vi "Do.vi"(8 "error in (no error)":errorcluster, 10 "Actor in":refnum<class "Actor.lvclass">, 11 "Set Ratios Msg":refnum<class "Set Ratios Msg.lvclass">) -> (0 "error out":errorcluster, 2 "Actor out":refnum<class "Actor.lvclass">)   [LabVIEW 2020, in "BNT_ULx.lvlib" / "Set Ratios Msg.lvclass"]
doc: "This VI delivers the message to the actor by calling the appropriate method(s) on the actor."
uses:
  Set Ratios Msg.lvclass
  <vilib>/ActorFramework/Actor/Actor.lvclass
  C:/User/Brand/LVP/CSPP/CSPP-Template/Packages/CSPP_Core/Messages/CSPP_PVUpdate Msg/CSPP_PVUpdate Msg.lvclass
  BNT_ULx-MCSV-DOPWM/BNT_ULx-MCSV-DOPWM.lvclass
  C:/Program Files (x86)/National Instruments/LabVIEW 2020/vi.lib/ActorFramework/Actor/Actor.lvclass
  CSPP_Core/Messages/CSPP_PVUpdate Msg/CSPP_PVUpdate Msg.lvclass/CSPP_PVUpdate Msg.ctl
  CSPP_Core/Classes/CSPP_ProcessVariables/ProcessVariable/PV.lvclass/PV.ctl
  Set Ratios Msg.lvclass/Set Ratios Msg.ctl
  CSPP_Core/Classes/CSPP_ProcessVariables/ProcessVariable/PV.lvclass
  CSPP_Core/Messages/CSPP_PVUpdate Msg/CSPP_PVUpdate Msg.lvclass
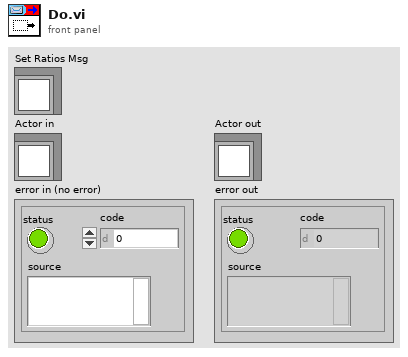
[diagram p1: front panel]
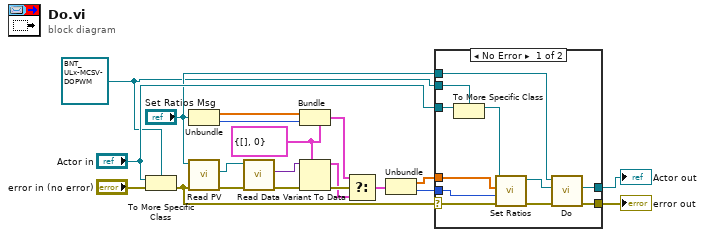
[diagram p0: block diagram]
diagram:
  w1 = refnum<class "BNT_ULx-MCSV-DOPWM.lvclass"> refnum ("BNT_ULx.lvlib:BNT_ULx-MCSV-DOPWM.lvclass")
  w14 = cluster{"PWM Ratios":dbl[], "Start Index":i32} {"PWM Ratios"=[], "Start Index"=0} ("Type")
  n1 = To More Specific Class(target class=w1, reference="Actor in", error in="error in (no error)") -> (error out=w11:errorcluster)  [unwired: 1 out]
  n2 = Unbundle ("Pre-Unbundler")("Set Ratios Msg") -> (w3:dbl[], w2:i32)
  n3 = call "Read PV.vi"("error in (no error)"=w11, "CS++PVUpdate Msg in"="Set Ratios Msg") -> ("error out"=w16:errorcluster, "PV"=w13:refnum<class "PV.lvclass">)  [unwired: 7 in, 1 out]
  n4 = call "Read Data.vi"("error in (no error)"=w16, "PV in"=w13) -> ("error out"=w7:errorcluster, "Data"=w6:variant)  [unwired: 7 in, 1 out]
  n5 = Bundle ("Pre-Bundler")(cluster=w14, "PWM Ratios"=w3, "Start Index"=w2) -> (w8:cluster{"PWM Ratios":dbl[], "Start Index":i32})
  n6 = Variant To Data(error in=w7, type=w14, Variant=w6) -> (data=w9:cluster{"PWM Ratios":dbl[], "Start Index":i32}, error out=w15:errorcluster)
  n7 = Select ("MainSelect")(t=w8, s=w15, f=w9) -> (s? t:f=w12:cluster{"PWM Ratios":dbl[], "Start Index":i32})
  n8 = Unbundle ("Main-Unbundler")(w12) -> ("PWM Ratios"=w5:dbl[], "Start Index"=w4:i32)
  n9 = case shown="No Error" w11 {
    selector: w11 -> [w23 w33]
    tunnel: [w28 w33] -> w19
    tunnel: [w29 w32] -> w18
    tunnel: "Actor in" -> [w31 w32]
    tunnel: w1 -> [w30 _]
    tunnel: "Set Ratios Msg" -> [w27 _]
    tunnel: w5 -> [w22 _]
    tunnel: w4 -> [w21 _]
    frame No Error {
      n10 = To More Specific Class ("To More Specific Class (internal)")(target class=w30, reference=w31) -> (specific class reference=w26:refnum<class "BNT_ULx-MCSV-DOPWM.lvclass">)  [unwired: 1 in, 1 out]
      n11 = call "Set Ratios.vi"("error in"=w23, "Start Index"=w21, "PWM Ratios"=w22, "BNT_ULx-MCSV-DOPWM in"=w26) -> ("error out"=w24:errorcluster, "BNT_ULx-MCSV-DOPWM out"=w25:refnum<class "BNT_ULx-MCSV-DOPWM.lvclass">)  [unwired: 6 in]
      n12 = call-parent "Do.vi"("error in (no error)"=w24, "Actor in"=w25, "CS++PVUpdate Msg"=w27) -> ("error out"=w28:errorcluster, "Actor out"=w29:refnum<class "Actor.lvclass">)  [unwired: 7 in]
    }
    frame Error {
    }
  }
  "error out" <- w19
  "Actor out" <- w18
